vi "Send Task Settings Payload.vi"(8 "error in (no error)":errorcluster, 10 "OK":bool, 11 "Task Setting Editor in":refnum<class "Task Setting Editor.lvclass">) -> (0 "error out":errorcluster, 3 "Task Setting Editor out":refnum<class "Task Setting Editor.lvclass">)   [LabVIEW 2017, in "Task Setting Editor.lvlib" / "Task Setting Editor.lvclass"]
uses:
  Task Setting Editor.lvclass
  <vilib>/ActorFramework/Stop Msg/Stop Msg.lvclass
  <vilib>/ActorFramework/Actor/Actor.lvclass
  BuildServer/BuildServer Messages/Update Tasks Msg/Update Tasks Msg.lvclass
  Volumes/Data/Users/benji667/Git/BuildFarm/WebSocket Server/Actors/Actor wHelper/Actor wHelper/Actor wHelper.lvclass
  Volumes/Data/Users/benji667/Git/BuildFarm/WebSocket Server/Actors/Actor wHelper/Actor wLauncher/Actor wLauncher.lvclass
  Volumes/Data/Users/benji667/Git/BuildFarm/WebSocket Server/Actors/Actor wHelper/Actor wUI/Actor wUI.lvclass
  Applications/National Instruments/LabVIEW 2017 64-bit/vi.lib/ActorFramework/Actor/Actor.lvclass
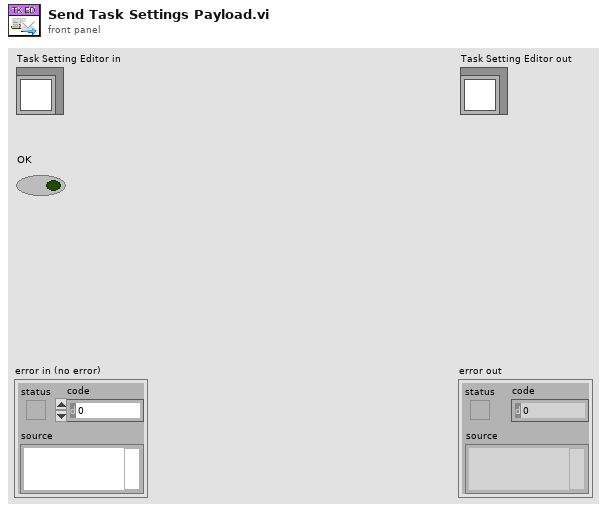
[diagram p1: front panel]
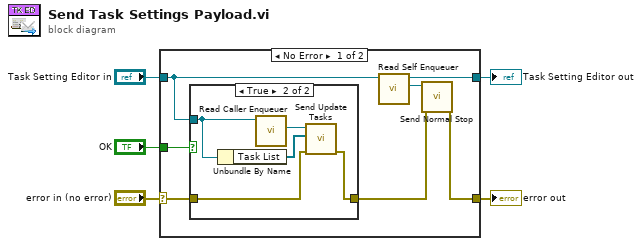
[diagram p0: block diagram]
diagram:
  n1 = case shown="No Error" "error in (no error)" {
    selector: "error in (no error)" -> [w11 w19]
    tunnel: [w6 w19] -> w4
    tunnel: [w9 w18] -> w2
    tunnel: "Task Setting Editor in" -> [w9 w18]
    tunnel: "OK" -> [w10 _]
    frame No Error {
      n2 = case shown="True" w10 {
        tunnel: w9 -> [_ w17]
        tunnel: w11 -> [w12 w14]
        tunnel: [w12 w13] -> w7
        frame False {
        }
        frame True {
          n3 = Unbundle By Name(w17) -> ("Task List"=w15:refnum<class "Task.lvclass">[])
          n4 = call <vilib>:"Read Caller Enqueuer.vi"("Actor"=w17) -> ("Caller Enqueuer"=w16:refnum<class "Message Enqueuer.lvclass">)  [unwired: 10 in]
          n5 = call "Send Update Tasks.vi"("error in (no error)"=w14, "Task List"=w15, "Message Enqueuer"=w16) -> ("error out"=w13:errorcluster)  [unwired: 7 in, 1 out]
        }
      }
      n6 = call <vilib>:"Read Self Enqueuer.vi"("Actor"=w9) -> ("Self Enqueuer"=w8:refnum<class "Message Enqueuer.lvclass">)  [unwired: 10 in]
      n7 = call <vilib>:"Send Normal Stop.vi"("error in (no error)"=w7, "Message Enqueuer"=w8) -> ("error out"=w6:errorcluster)  [unwired: 9 in]
    }
    frame Error {
    }
  }
  "error out" <- w4
  "Task Setting Editor out" <- w2
